vi "Read Query Result.vi"(8 "error in (no error)":errorcluster, 11 ".NET Refnum in":refnum<k24>) -> (0 "error out":errorcluster, 2 "Data":string[][](array[string]), 3 ".NET Refnum out":refnum<k24>)   [LabVIEW 2017, in "VIs to Interface LabVIEW and MySQL dotNET Connector.lvlib"]
doc: "Read data returned by a query command."
uses:
  VIs to Interface LabVIEW and MySQL dotNET Connector.lvlib
  MySql.Data
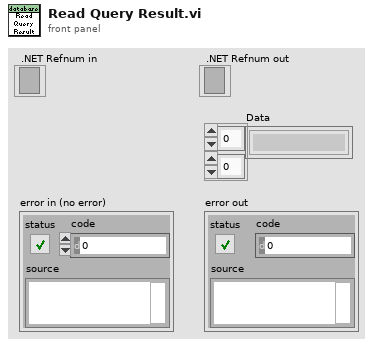
[diagram p1: front panel]
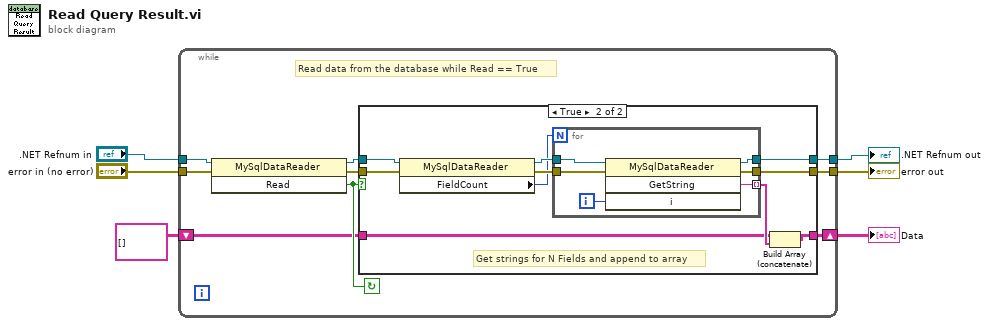
[diagram p0: block diagram]
diagram:
  n1 = while {
    tunnel: ".NET Refnum in" -> [w15]
    tunnel: "error in (no error)" -> [w14]
    tunnel: [w13] -> w3
    tunnel: [w12] -> w4
    shift-right: [w11] -> w5
    shift-left: string[][] [] -> [w7]
    stop <- w8 continue-if-true
    # "Read data from the database while Read == True"
    n2 = invoke class="MySqlDataReader" method="Read"(reference=w15, error in=w14) -> (reference out=w10:refnum<k24>, error out=w9:errorcluster, "Read"=w8:bool)  [unwired: 1 in]
    n3 = case shown="True" w8 {
      tunnel: [w18 w28] -> w13
      tunnel: [w17 w27] -> w12
      tunnel: [w16 w20] -> w11
      tunnel: w10 -> [w18 w25]
      tunnel: w9 -> [w17 w24]
      tunnel: w7 -> [w16 w19]
      frame False {
        # "Read complete"
      }
      frame True {
        # "Get strings for N Fields and append to array"
        n4 = property class="MySqlDataReader"(reference=w25, error in=w24) -> (reference out=w23:refnum<k24>, error out=w22:errorcluster, "FieldCount"=w21:i32)
        n5 = for {
          N: w21 -> [_]
          tunnel: [w34] -> w28
          tunnel: [w33] -> w27
          tunnel: [w32] -> w26 mode=indexing
          tunnel: w23 -> [w31]
          tunnel: w22 -> [w30]
          i -> [w29]
          n6 = invoke class="MySqlDataReader" method="GetString"(reference=w31, error in=w30, "i"=w29) -> (reference out=w34:refnum<k24>, error out=w33:errorcluster, "GetString"=w32:string)  [unwired: 1 in, 1 out]
        }
        n7 = Build Array (concatenate)(w19, w26) -> (w20:string[][])
      }
    }
  }
  "Data" <- w5
  "error out" <- w4
  ".NET Refnum out" <- w3
